vi "p_meas_measure.vi"(7 "Samples":i32=5, 8 "error out 2":errorcluster, 10 "Boolean":bool, 11 "dup Visa Session":refnum<visa-resource-name>) -> (0 "error out":errorcluster, 1 "variance":dbl format="%.2e", 2 "std deviation":dbl format="%.2e", 3 "mean":dbl format="%.2e", 5 "dup Visa Session 2":refnum<visa-resource-name>)   [LabVIEW 2012]
doc: "PowerDemo.vi\nThe Demo enables power measurement and display results.\nVersion 1.00\nLast Updated 16 Mars 2005\n\nDemo Program Steps:\n \n1) The vi executes InitCom.vi to open the communication session.\nThe default is RS232,Port2,9600 bps and Address 10 for USB.\n\nYou have to select USB or RS232 Protocol and\nupdate these values for any change.\n\n2) The vi executes ConfMeasure.vi to Send \"FP\" (Force Power) to Device and \"SI\" (Send unIts) to receive the units\n\n3) The vi executes a loop of SendPower.vi to get measurements.\nWhen no Overrange value the vi add value to array for update\nstatistics values.\n\nIn case of Error:\nError Out contains the Error Number and the vi's name where the error occured.\n\nVISA Error Codes -10738077360 to -1073807231\nOphir Error Codes -1300 to 1340"
uses:
  <vilib>/Analysis/NI_AALBase.lvlib
panel:
  out "Overrange":bool
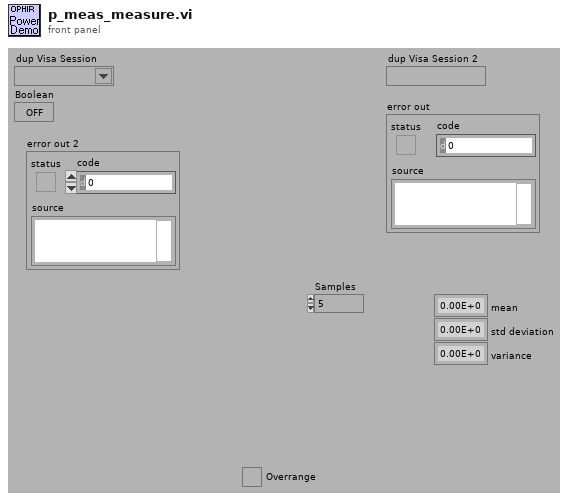
[diagram p1: front panel]
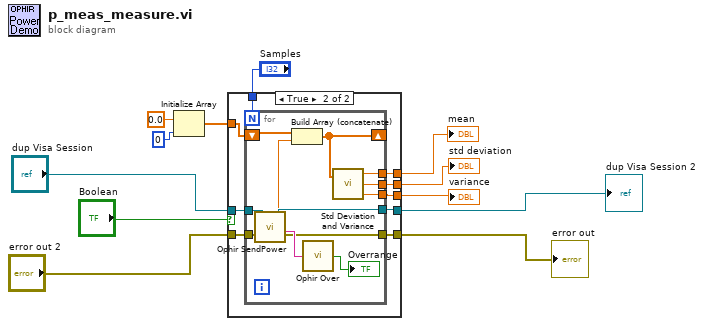
[diagram p0: block diagram]
diagram:
  n1 = Initialize Array(0.0 ("element"), 0 ("dimension size")) -> (w7:dbl[])
  n2 = case shown="True" "Boolean" {
    tunnel: "dup Visa Session" -> [w13 w23]
    tunnel: "error out 2" -> [w14 w22]
    tunnel: [w13 w21] -> w12
    tunnel: [w14 w20] -> w11
    tunnel: "Samples" -> [_ w19]
    tunnel: w7 -> [_ w18]
    tunnel: [_ w17] -> w6
    tunnel: [_ w16] -> w5
    tunnel: [_ w15] -> w4
    frame False {
      # "Force Power Configuration failed"
    }
    frame True {
      n3 = for {
        N: w19 -> [_]
        tunnel: w23 -> [w35]
        tunnel: w22 -> [w34]
        tunnel: [w33] -> w21
        tunnel: [w30] -> w20
        shift-right: [w27] -> _
        shift-left: w18 -> [w29]
        tunnel: [w26] -> w15
        tunnel: [w25] -> w16
        tunnel: [w24] -> w17
        n4 = call "Ophir SendPower.vi"("Visa Session"=w35, "error in (no error)"=w34) -> ("dup Visa Session"=w33:refnum<visa-resource-name>, "Value Number"=w28:dbl, "Value String"=w32:string, "error out"=w30:errorcluster)
        n5 = Build Array (concatenate)(w29, w28) -> (w27:dbl[])
        n6 = call "Ophir Over.vi"("Value String"=w32) -> ("Overrange"=→"Overrange":bool)
        n7 = call <vilib>:"Std Deviation and Variance.vi"("X"=w27) -> ("mean"=w26:dbl, "standard deviation"=w25:dbl, "variance"=w24:dbl)  [unwired: 1 in]
      }
    }
  }
  "mean" <- w4
  "std deviation" <- w5
  "variance" <- w6
  "dup Visa Session 2" <- w12
  "error out" <- w11
